vi "E7_28.vi"(4 "error in":T15, 7 "Command":T7) -> (0 "error out":T15, 3 "Response":T13)   [LabVIEW 2018]
uses:
  MOKO_LabViewLibrary/MokoLowLevel/MokoLowLovelControl/MLLC_Command.ctl
  MOKO_LabViewLibrary/MokoLowLevel/MokoLowLovelControl/MLLC_Error.ctl
  MOKO_LabViewLibrary/MokoLowLevel/MokoLowLovelControl/MLLC_Mode.ctl
  MOKO_LabViewLibrary/MokoLowLevel/MokoLowLovelControl/MLLC_Response.ctl
  MOKO_LabViewLibrary/MokoLowLevel/MokoLowLovelControl/MLLC_DriverName.ctl
  MOKO_LabViewLibrary/MokoLowLevel/MokoLowLovelControl/MLLC_ResponseInit.ctl
  MOKO_LabViewLibrary/MokoLowLevel/MokoLowLovelControl/MLLC_ErrorCode.ctl
  MOKO_LabViewLibrary/MokoLowLevel/MokoLowLovelControl/MLLC_Request.ctl
  MOKO_LabViewLibrary/MokoLowLevel/MokoLowLovelControl/MLLC_ConnectCluster.ctl
  MOKO_LabViewLibrary/MokoLowLevel/MokoLowLovelControl/MLLC_InterfaceType.ctl
  MOKO_LabViewLibrary/MokoLowLevel/MokoLowLovelControl/MLLC_OpenedSession.ctl
  MOKO_LabViewLibrary/MokoLowLevel/MokoLowLovelControl/MLLC_InterfaceSettings.ctl
  MOKO_LabViewLibrary/MokoLowLevel/MokoLowLovelControl/MLLC_InterfaceKind.ctl
  data/E7_28_DATA.ctl
  MOKO_LabViewLibrary/MokoLowLevel/MokoLowLovelControl/MLLC_Rs232Settings.ctl
panel:
  in  "Settings":T9={"Data"={"Connect"={"InterfaceType"=enum."VISA", "OpenedSession"="", "InterfaceSettings"={"Interface"=enum."RS232", "EOS 4 read"=enum."LF (\\n)", "EOS 4 write"=enum."LF (\\n)", "TMO, ms"=10000, "Sett"=variant(cluster{"Baud Rate":u32, "Data Bits":u16, "Parity":u16, "Stop Bits":u16, "Flow Control":u16, "Eho":bool} {"Baud Rate"=75, "Data Bits"=0, "Parity"=0, "Stop Bits"=0, "Flow Control"=0, "Eho"=FALSE})}}, "Cluster"={"flags"="", "freq"=0, "z"=0.0, "f"=0}, "Delay, ms"=100}, "Saved Data"=variant}
  in  "Request":T10="init"
  in  "Error Code":T8=5422
  in  "ResponseInit":T11="Є@E728"
  in  "Driver Name":T12="E7_28"
  in  "Mode":T14=enum."Check"
  # "E7-28"
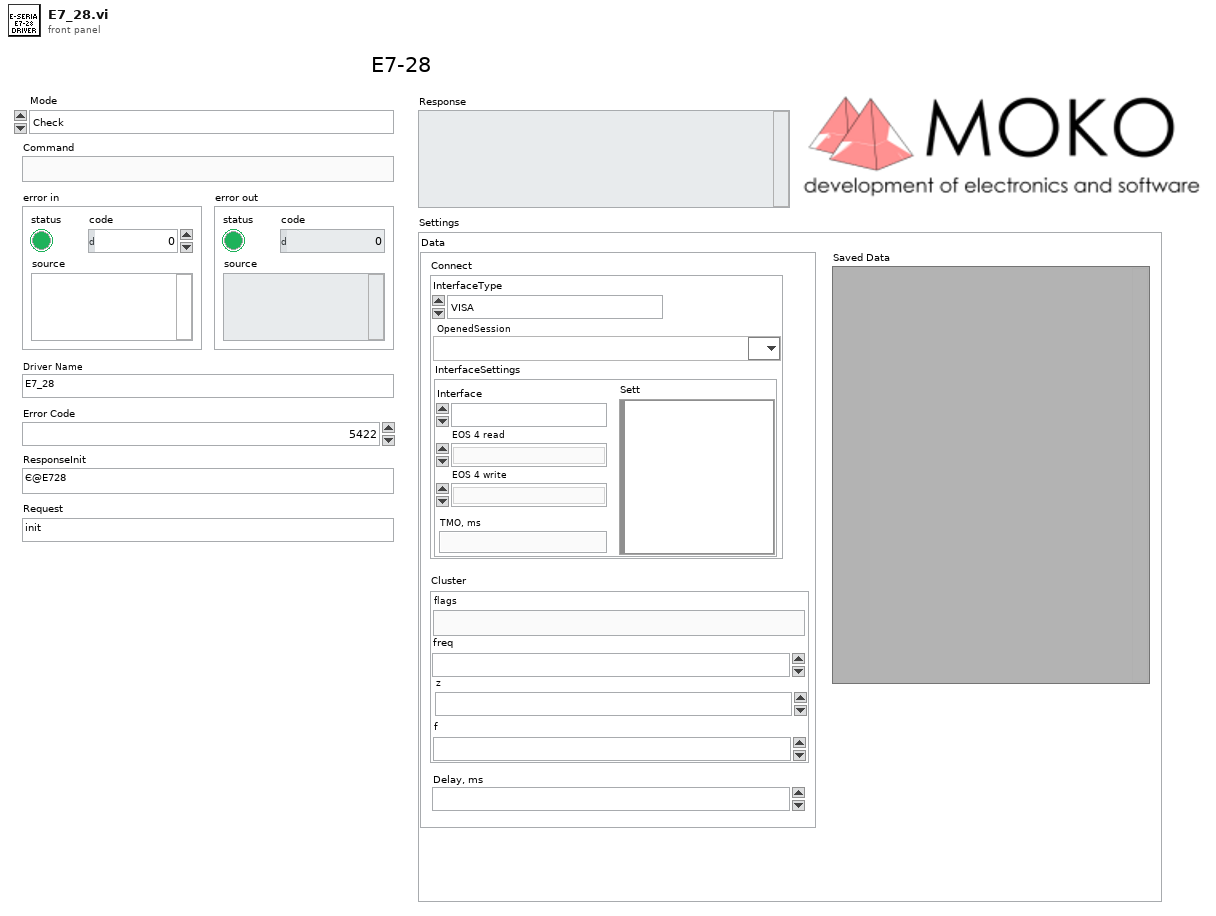
[diagram p1: front panel]
types:
  T1 = typedef "MLLC_ConnectCluster.ctl" = cluster{"InterfaceType":T2, "OpenedSession":T3, "InterfaceSettings":T4}
  T2 = typedef "MLLC_InterfaceType.ctl" = enum16{"VISA", "Prologix USB-GPIB"}
  T3 = typedef "MLLC_OpenedSession.ctl" = refnum<visa-resource-name>
  T4 = typedef "MLLC_InterfaceSettings.ctl" = cluster{"Interface":T5, "EOS 4 read":enum16{"Default (=EOS 4 write)", "CR (\\r)", "LF (\\n)", "None"}, "EOS 4 write":enum16{"CR+LF (\\r\\n)", "CR (\\r)", "LF (\\n)", "None"}, "TMO, ms":i32, "Sett":variant}
  T5 = typedef "MLLC_InterfaceKind.ctl" = enum16{"RS232", "GPIB", "USB", "Ethernet", "another"}
  T6 = typedef "E7_28_DATA.ctl" = cluster{"flags":T7, "freq":T8, "z":dbl, "f":T8}
  T7 = typedef "MLLC_Command.ctl" = string
  T8 = typedef "MLLC_ErrorCode.ctl" = u32
  T9 = cluster{"Data":cluster{"Connect":T1, "Cluster":T6, "Delay, ms":T8}, "Saved Data":variant}
  T10 = typedef "MLLC_Request.ctl" = string
  T11 = typedef "MLLC_ResponseInit.ctl" = string
  T12 = typedef "MLLC_DriverName.ctl" = string
  T13 = typedef "MLLC_Response.ctl" = string
  T14 = typedef "MLLC_Mode.ctl" = enum16{"get", "set", "close", "Init", "Check"}
  T15 = typedef "MLLC_Error.ctl" = errorcluster
  T16 = cluster{"Connect":T1, "Cluster":T6, "Delay, ms":T8}
  T17 = typedef "MLLC_Rs232Settings.ctl" = cluster{"Baud Rate":u32, "Data Bits":u16, "Parity":u16, "Stop Bits":u16, "Flow Control":u16, "Eho":bool, "Address":dbl}
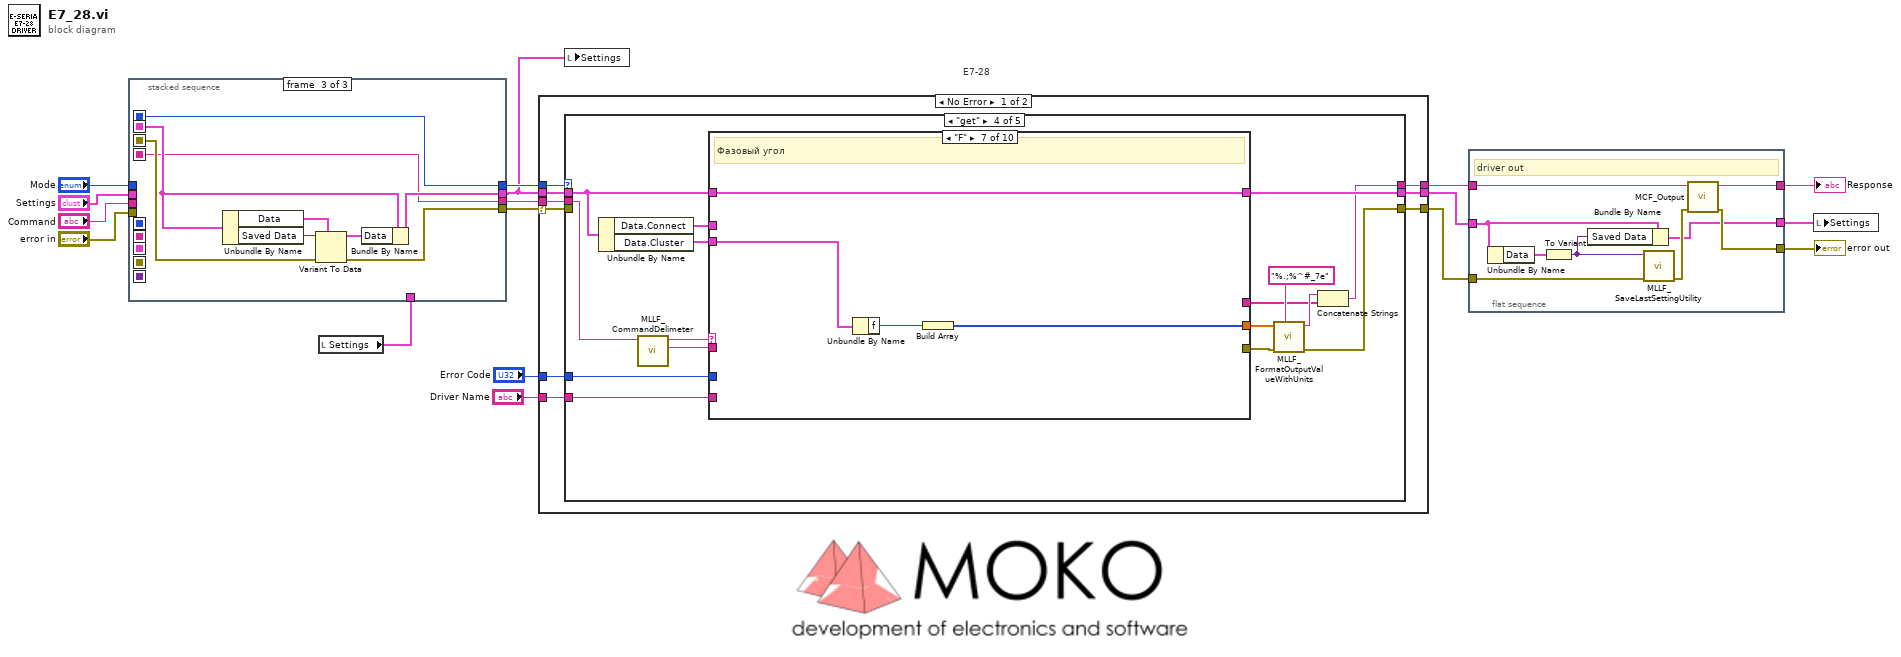
[diagram p0: block diagram]
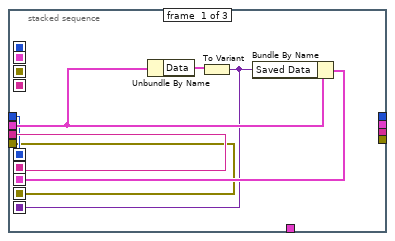
[diagram p2: hidden frame]
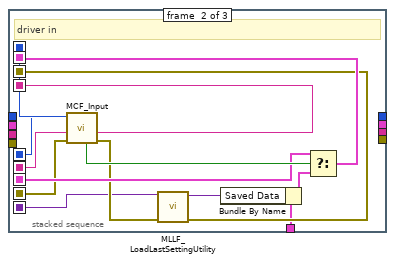
[diagram p3: hidden frame]
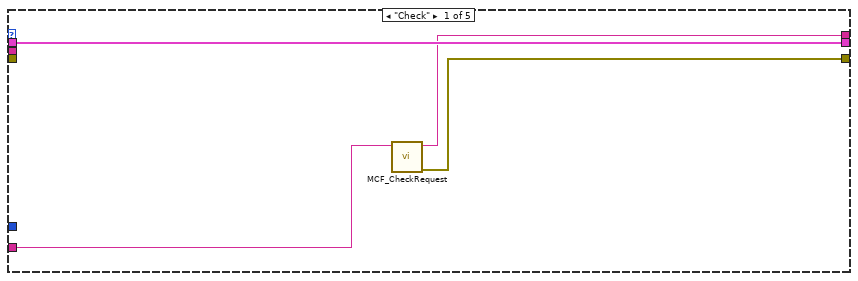
[diagram p4: hidden frame]
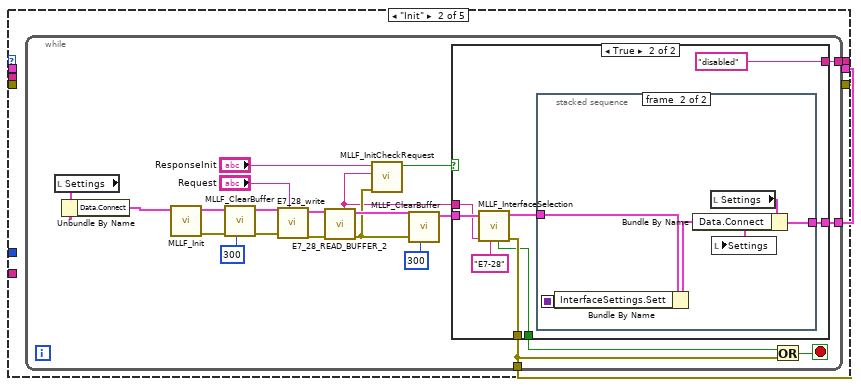
[diagram p5: hidden frame]
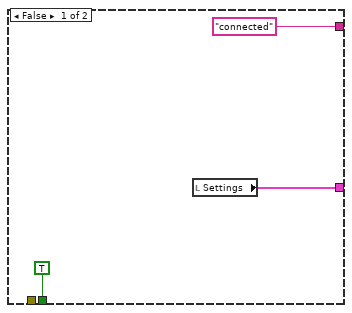
[diagram p6: hidden frame]
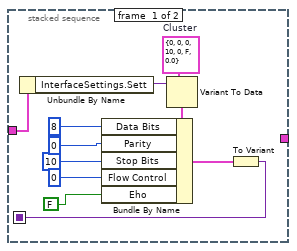
[diagram p7: hidden frame]
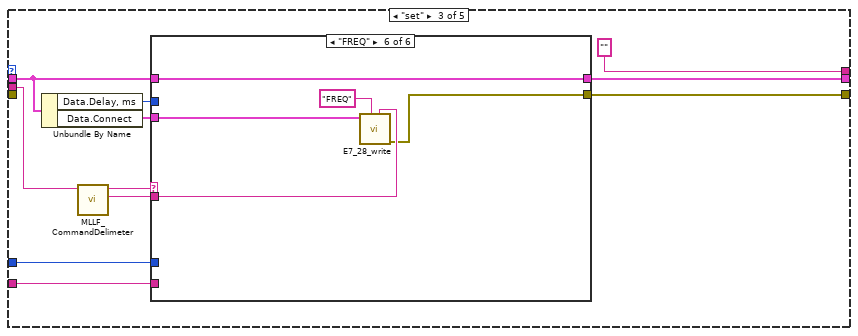
[diagram p8: hidden frame]
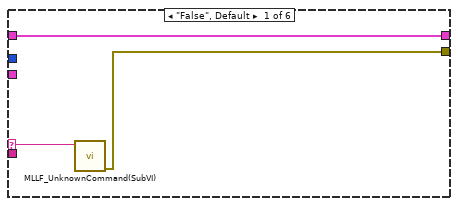
[diagram p9: hidden frame]
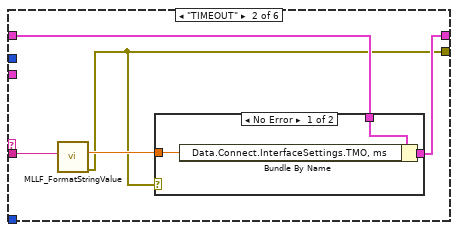
[diagram p10: hidden frame]
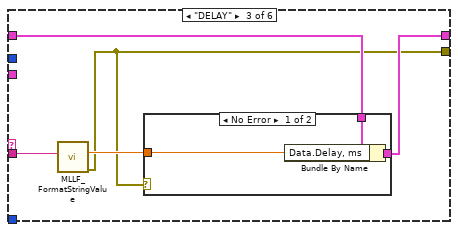
[diagram p12: hidden frame]
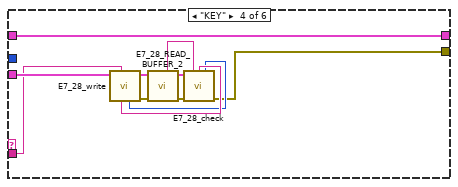
[diagram p14: hidden frame]
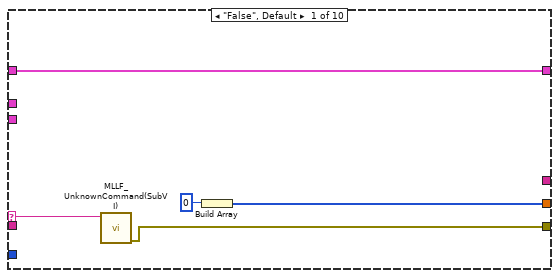
[diagram p16: hidden frame]
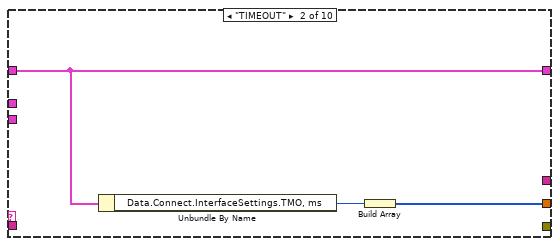
[diagram p17: hidden frame]
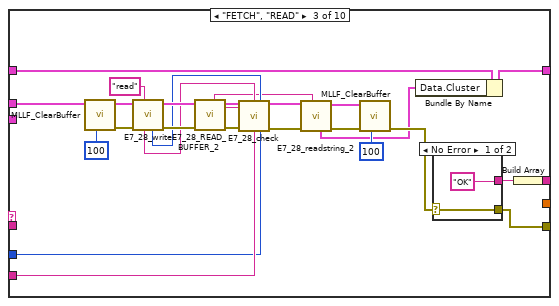
[diagram p18: hidden frame]
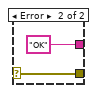
[diagram p19: hidden frame]
diagram:
  # "E7-28"
  n1 = local read "Settings"() -> (w7:T9)
  n2 = stacked-sequence {
    seq-local: [w20 _ _] -> [_ w36 _]
    seq-local: [w19 _ _] -> [_ w37 _]
    seq-local: [w22 _ _] -> [_ w32 _]
    seq-local: [w18 _ _] -> [_ w31 _]
    seq-local: [w21 _ _] -> [_ w27 _]
    seq-local: [_ w28 _] -> [_ _ w44]
    seq-local: [_ w38 _] -> [_ _ w41]
    seq-local: [_ w35 _] -> [_ _ w40]
    seq-local: [_ w34 _] -> [_ _ w45]
    tunnel: "Command" -> [w20 _ _]
    tunnel: "Mode" -> [w19 _ _]
    tunnel: "error in" -> [w18 _ _]
    tunnel: "Settings" -> [w23 _ _]
    tunnel: w7 -> [_ w26 _]
    tunnel: [_ _ w40] -> w9
    tunnel: [_ _ w43] -> w10
    tunnel: [_ _ w42] -> w8
    tunnel: [_ _ w41] -> w11
    frame #0 {
      n3 = Unbundle By Name(w23) -> ("Data"=w24:T16)
      n4 = To Variant(anything=w24) -> (Variant=w21:variant)
      n5 = Bundle By Name(cluster=w23, "Saved Data"=w21) -> (w22:T9)
    }
    frame #1 {
      # "driver in"
      n6 = call "MCF_Input.vi"("Error In"=w31, "Command in"=w36, "Mode in"=w37) -> ("Error Out"=w30:errorcluster, "Command out"=w35:string, "Mode out"=w38:T14, "Boolean"=w33:bool)  [unwired: 5 in]
      n7 = call "MLLF_LoadLastSettingUtility.vi"("Error In"=w30, "Save data in"=w27) -> ("Error Out"=w28:errorcluster, "Save data out"=w25:variant)  [unwired: 8 in]
      n8 = Bundle By Name(cluster=w26, "Saved Data"=w25) -> (w29:T9)
      n9 = Select(t=w32, s=w33, f=w29) -> (s? t:f=w34:T9)
    }
    frame #2 {
      n10 = Unbundle By Name(w45) -> ("Data"=w46:T16, "Saved Data"=w39:variant)
      n11 = Variant To Data(error in=w44, type=w46, Variant=w39) -> (data=w47:T16, error out=w42:errorcluster)
      n12 = Bundle By Name(cluster=w45, "Data"=w47) -> (w43:T9)
    }
  }
  n13 = case shown="No Error" w8 {
    selector: w8 -> [w52 w267]
    tunnel: [w54 w267] -> w4
    tunnel: w11 -> [w56 _]
    tunnel: [w55 "" ("String")] -> w6
    tunnel: w9 -> [w53 _]
    tunnel: w10 -> [w49 w266]
    tunnel: "Error Code" -> [w51 _]
    tunnel: "Driver Name" -> [w50 _]
    tunnel: [w48 w266] -> w5
    frame No Error {
      n14 = case shown="\"get\"" w56 {
        tunnel: [w59 w63 "" ("String") w163 _] -> w55
        tunnel: [w58 w61 w113 w162 w263] -> w54
        tunnel: w53 -> [_ _ w116 w166 _]
        tunnel: w52 -> [_ _ _ _ _]
        tunnel: w51 -> [_ _ w123 w175 _]
        tunnel: w50 -> [w57 _ w120 w174 _]
        tunnel: w49 -> [w60 _ w122 w177 w262]
        tunnel: [w60 w62 w121 w176 w262] -> w48
        frame "Check" {
          n15 = call "MCF_CheckRequest.vi"("Driver Name"=w57) -> ("Error Out"=w58:errorcluster, "Output String"=w59:string)  [unwired: 9 in]
        }
        frame "Init" {
          n16 = while {
            tunnel: [w83] -> w61
            tunnel: [w66] -> w63
            tunnel: [w65] -> w62
            stop <- w82 stop-if-true
            n17 = local read "Settings"() -> (w85:T9)
            n18 = Unbundle By Name(w85) -> ("Data.Connect"=w84:T1)
            n19 = call "MLLF_Init.vi"("DriverConnect in"=w84) -> ("Error Out"=w77:errorcluster, "DriverConnect out"=w78:T1)  [unwired: 7 in]
            n20 = call "MLLF_ClearBuffer.vi"("Timeout(default = 300 ms)"=u32 300 ("Timeout"), "Error In"=w77, "DriverConnect in"=w78) -> ("Error Out"=w75:errorcluster, "DriverConnect out"=w76:T1)  [unwired: 5 in, 1 out]
            n21 = call "E7_28_write.vi"("Command"="Request", "error in"=w75, "DriverConnect in"=w76) -> ("error out"=w80:T15, "DriverConnect out"=w79:T1)  [unwired: 5 in, 2 out]
            n22 = call "E7_28_READ_BUFFER_2.vi"("error in"=w80, "DriverConnect in"=w79) -> ("error out"=w69:T15, "DriverConnect out"=w72:T1, "String from device out"=w64:string)  [unwired: 7 in]
            n23 = call "MLLF_InitCheckRequest.vi"("error in (no error)"=w69, "Answer"=w64, "Response Init"="ResponseInit") -> ("Design"=w68:bool)  [unwired: 5 in, 3 out]
            n24 = call "MLLF_ClearBuffer.vi"("Timeout(default = 300 ms)"=u32 300 ("Timeout"), "Error In"=w69, "DriverConnect in"=w72) -> ("DriverConnect out"=w71:T1)  [unwired: 5 in, 2 out]
            n25 = case shown="True" w68 {
              tunnel: [_ w94] -> w83
              tunnel: [TRUE w90] -> w81
              tunnel: w71 -> [_ w96]
              tunnel: ["connected" "disabled"] -> w66
              tunnel: [w86 w91] -> w65
              tunnel: w64 -> [_ w89]
              frame False {
                n26 = local read "Settings"() -> (w86:T9)
              }
              frame True {
                n27 = call "MLLF_InterfaceSelection.vi"("Driver Name"="E7-28" ("String"), "Answer:"=w89, "DriverConnect in"=w96) -> ("error out"=w94:T15, "DriverConnect out"=w95:T1, "stop init?"=w90:bool)  [unwired: 4 in, 2 out]
                n28 = stacked-sequence {
                  seq-local: [w99 _] -> [_ w111]
                  tunnel: w95 -> [w97 w109]
                  tunnel: [_ w110] -> w91
                  frame #0 {
                    w106 = T17 {"Baud Rate"=0, "Data Bits"=0, "Parity"=0, "Stop Bits"=10, "Flow Control"=0, "Eho"=FALSE, "Address"=0.0}  # Cluster
                    n29 = Unbundle By Name(w97) -> ("InterfaceSettings.Sett"=w107:variant)
                    n30 = Variant To Data(type=w106, Variant=w107) -> (data=w105:T17)  [unwired: 1 in, 1 out]
                    n31 = Bundle By Name(cluster=w105, "Data Bits"=u16 8 ("Serial Settings:Data Bits"), "Parity"=u16 0 ("Serial Settings:Parity"), "Stop Bits"=u16 10 ("Serial Settings:Stop Bits"), "Flow Control"=u16 0 ("Serial Settings:Flow Control"), "Eho"=FALSE) -> (w100:T17)
                    n32 = To Variant(anything=w100) -> (Variant=w99:variant)
                  }
                  frame #1 {
                    n33 = Bundle By Name(cluster=w109, "InterfaceSettings.Sett"=w111) -> (w108:T1)
                    n34 = local read "Settings"() -> (w112:T9)
                    n35 = Bundle By Name(cluster=w112, "Data.Connect"=w108) -> (w110:T9)
                    n36 = local write "Settings"(w110) -> ()
                  }
                }
              }
            }
            n37 = Or(x=w81, y=w83) -> (x .or. y?=w82:bool)
          }
        }
        frame "set" {
          n38 = Unbundle By Name(w122) -> ("Data.Delay, ms"=w117:T8, "Data.Connect"=w118:T1)
          n39 = call "MLLF_CommandDelimeter.vi"("command with param"=w116) -> ("param 1"=w114:string, "command"=w115:string)  [unwired: 6 in, 3 out]
          n40 = case shown="\"FREQ\"" w115 {
            selector: w115 -> [w125 _ _ _ _ _]
            tunnel: w114 -> [_ w129 w138 w153 _ w158]
            tunnel: [w124 w127 w136 w145 _ w157] -> w113
            tunnel: w123 -> [_ _ _ _ _ _]
            tunnel: w122 -> [w126 w130 w139 w155 w156 w161]
            tunnel: [w126 w131 w140 w155 w156 w161] -> w121
            tunnel: w118 -> [_ _ _ w154 _ w160]
            tunnel: w120 -> [_ _ _ _ _ _]
            tunnel: w117 -> [_ _ _ _ _ _]
            frame "False", Default {
              n41 = call "MLLF_UnknownCommand(SubVI).vi"("Unknown command"=w125) -> ("error out"=w124:errorcluster)  [unwired: 10 in]
            }
            frame "TIMEOUT" {
              n42 = call "MLLF_FormatStringValue.vi"("String Value"=w129) -> ("error out"=w127:T15, "number"=w128:dbl)  [unwired: 8 in, 1 out]
              n43 = case shown="No Error" w127 {
                tunnel: [w134 w135] -> w131
                tunnel: w130 -> [w133 w135]
                tunnel: w128 -> [w132 _]
                frame No Error {
                  n44 = Bundle By Name(cluster=w133, "Data.Connect.InterfaceSettings.TMO, ms"=w132) -> (w134:T9)
                }
                frame Error {
                }
              }
            }
            frame "DELAY" {
              n45 = call "MLLF_FormatStringValue.vi"("String Value"=w138) -> ("error out"=w136:T15, "number"=w137:dbl)  [unwired: 8 in, 1 out]
              n46 = case shown="No Error" w136 {
                tunnel: [w143 w144] -> w140
                tunnel: w139 -> [w142 w144]
                tunnel: w137 -> [w141 _]
                frame No Error {
                  n47 = Bundle By Name(cluster=w142, "Data.Delay, ms"=w141) -> (w143:T9)
                }
                frame Error {
                }
              }
            }
            frame "KEY" {
              n48 = call "E7_28_write.vi"("Command"=w153, "DriverConnect in"=w154) -> ("error out"=w149:T15, "DriverConnect out"=w150:T1, "command HEX out"=w147:u16, "command string out"=w148:T7)  [unwired: 6 in]
              n49 = call "E7_28_READ_BUFFER_2.vi"("error in"=w149, "DriverConnect in"=w150) -> ("error out"=w151:T15, "DriverConnect out"=w152:T1, "String from device out"=w146:string)  [unwired: 7 in]
              n50 = call "E7_28_check.vi"("DriverConnect in"=w152, "String in"=w146, "command string in"=w148, "command HEX in"=w147, "error in"=w151) -> ("error out"=w145:T15)  [unwired: 9 in, 1 out]
            }
            frame "---------------------------------------------------------------------------------------" {
            }
            frame "FREQ" {
              n51 = call "E7_28_write.vi"("VALUE"=w158, "Command"="FREQ", "DriverConnect in"=w160) -> ("error out"=w157:T15)  [unwired: 5 in, 3 out]
            }
          }
        }
        frame "get" {
          n52 = Unbundle By Name(w177) -> ("Data.Connect"=w170:T1, "Data.Cluster"=w167:T6)
          n53 = call "MLLF_CommandDelimeter.vi"("command with param"=w166) -> ("param 1"=w164:string, "command"=w165:string)  [unwired: 6 in, 3 out]
          n54 = case shown="\"F\"" w165 {
            selector: w165 -> [w179 _ _ _ _ _ _ _ _ _]
            tunnel: w164 -> [_ _ _ _ _ _ _ _ _ _]
            tunnel: [w178 _ w195 _ _ _ _ _ _ _] -> w172
            tunnel: w175 -> [_ _ w200 _ _ _ _ _ _ _]
            tunnel: [w182 w185 w187 w216 w217 w221 w225 w234 w244 w256] -> w176
            tunnel: [w180 w183 _ _ w218 w222 w226 w236 w245 w257] -> w171
            tunnel: w170 -> [_ _ w205 _ _ _ _ _ _ _]
            tunnel: w174 -> [_ _ w201 _ _ _ _ _ _ _]
            tunnel: [_ _ w196 _ _ _ _ _ _ _] -> w168
            tunnel: w167 -> [_ _ _ _ w220 w224 w228 w240 w246 w259]
            tunnel: w177 -> [w182 w185 w188 w216 w217 w221 w225 w234 w244 w256]
            frame "False", Default {
              n55 = call "MLLF_UnknownCommand(SubVI).vi"("Unknown command"=w179) -> ("error out"=w178:errorcluster)  [unwired: 10 in]
              n56 = Build Array(0 ("TimeOut")) -> (w180:i32[])
            }
            frame "TIMEOUT" {
              n57 = Unbundle By Name(w185) -> ("Data.Connect.InterfaceSettings.TMO, ms"=w184:i32)
              n58 = Build Array(w184) -> (w183:i32[])
            }
            frame "FETCH", "READ" {
              n59 = call "MLLF_ClearBuffer.vi"("Timeout(default = 300 ms)"=u32 100 ("Timeout"), "DriverConnect in"=w205) -> ("Error Out"=w208:errorcluster, "DriverConnect out"=w209:T1)  [unwired: 6 in, 1 out]
              n60 = call "E7_28_write.vi"("Command"="read", "error in"=w208, "DriverConnect in"=w209) -> ("error out"=w211:T15, "DriverConnect out"=w210:T1, "command HEX out"=w198:u16, "command string out"=w199:T7)  [unwired: 5 in]
              n61 = call "E7_28_READ_BUFFER_2.vi"("error in"=w211, "DriverConnect in"=w210) -> ("error out"=w202:T15, "DriverConnect out"=w203:T1, "String from device out"=w192:string)  [unwired: 7 in]
              n62 = call "E7_28_check.vi"("DriverConnect in"=w203, "String in"=w192, "command string in"=w199, "command HEX in"=w198, "error in"=w202, "Driver Name"=w201, "Error Code"=w200) -> ("DriverConnect out"=w194:T1, "error out"=w193:T15)  [unwired: 7 in]
              n63 = call "E7_28_readstring_2.vi"("data string"=w192, "error in"=w193, "DriverConnect in"=w194) -> ("error out"=w190:T15, "DriverConnect out"=w191:T1, "Cluster 2"=w186:T6)  [unwired: 6 in]
              n64 = call "MLLF_ClearBuffer.vi"("Timeout(default = 300 ms)"=u32 100 ("Timeout"), "Error In"=w190, "DriverConnect in"=w191) -> ("Error Out"=w189:errorcluster)  [unwired: 5 in, 2 out]
              n65 = Bundle By Name(cluster=w188, "Data.Cluster"=w186) -> (w187:T9)
              n66 = case shown="No Error" w189 {
                selector: w189 -> [w213 w214]
                tunnel: [w213 w214] -> w195
                tunnel: ["OK" "OK"] -> w197
                frame No Error {
                }
                frame Error {
                }
              }
              n67 = Build Array(w197) -> (w196:string[])
            }
            frame "---------------------------------------------------------" {
            }
            frame "FREQ" {
              n68 = Unbundle By Name(w220) -> ("freq"=w219:T8)
              n69 = Build Array(w219) -> (w218:T8[])
            }
            frame "Z" {
              # "Модуль комплексного сопротивления, Z"
              n70 = Unbundle By Name(w224) -> ("z"=w223:dbl)
              n71 = Build Array(w223) -> (w222:dbl[])
            }
            frame "F" {
              # "Фазовый угол"
              n72 = Unbundle By Name(w228) -> ("f"=w227:T8)
              n73 = Build Array(w227) -> (w226:T8[])
            }
            frame "C" {
              # "Емкость С, Ф"
              n74 = Unbundle By Name(w240) -> ("freq"=w239:T8)
              n75 = Unbundle By Name(w240) -> ("z"=w243:dbl)
              n76 = Unbundle By Name(w240) -> ("f"=w230:T8)
              n77 = Divide(x=w230, y=57.2958) -> (x/y=w231:dbl)
              n78 = Sine(x=w231) -> (sin(x)=w242:dbl)
              n79 = Multiply(x=w243, y=w242) -> (x*y=w241:dbl)
              n80 = Multiply(x=w239, y=6.283185307179586) -> (x*y=w237:dbl)
              n81 = Multiply(x=w241, y=w237) -> (x*y=w235:dbl)
              n82 = Reciprocal(x=w235) -> (1/x=w233:dbl)
              n83 = Absolute Value(x=w233) -> (abs(x)=w232:dbl)
              n84 = Build Array(w232) -> (w236:dbl[])
            }
            frame "R", "Rs" {
              n85 = Unbundle By Name(w246) -> ("z"=w253:dbl)
              n86 = Unbundle By Name(w246) -> ("f"=w248:T8)
              n87 = Divide(x=w248, y=57.2958) -> (x/y=w247:dbl)
              n88 = Absolute Value(x=w253) -> (abs(x)=w252:dbl)
              n89 = Cosine(x=w247) -> (cos(x)=w251:dbl)
              n90 = Multiply(x=w252, y=w251) -> (x*y=w250:dbl)
              n91 = Build Array(w250) -> (w245:dbl[])
            }
            frame "D" {
              # "Фактор потерь, D"
              n92 = Unbundle By Name(w259) -> ("f"=w261:T8)
              n93 = Divide(x=w261, y=57.2958) -> (x/y=w258:dbl)
              n94 = Tangent(1:w258) -> (0:w255:dbl)
              n95 = Absolute Value(x=w255) -> (abs(x)=w254:dbl)
              n96 = Build Array(w254) -> (w257:dbl[])
            }
          }
          n97 = call "MLLF_FormatOutputValueWithUnits.vi"("Format"="%.;%^#_7e" ("format string"), "error in"=w172, "ValuesIn"=w171) -> ("error out"=w162:T15, "Result string"=w173:T7)  [unwired: 7 in]
          n98 = Concatenate Strings(w173, w168) -> (w163:string)
        }
        frame "close" {
          n99 = Unbundle By Name(w262) -> ("Data.Connect.OpenedSession"=w264:T3)
          n100 = VISA Close(VISA resource name=w264) -> (error out=w263:errorcluster)  [unwired: 1 in]
        }
      }
    }
    frame Error {
    }
  }
  n101 = local write "Settings"(w10) -> ()
  n102 = flat-sequence {
    tunnel: [w276] -> w3
    tunnel: [w275] -> w1
    tunnel: w6 -> [w274]
    tunnel: w4 -> [w273]
    tunnel: w5 -> [w270]
    tunnel: [w268] -> _
    tunnel: [w268] -> w2
    frame #0 {
      # "driver out"
      n103 = Unbundle By Name(w270) -> ("Data"=w269:T16)
      n104 = To Variant(anything=w269) -> (Variant=w271:variant)
      n105 = Bundle By Name(cluster=w270, "Saved Data"=w271) -> (w268:T9)
      n106 = call "MLLF_SaveLastSettingUtility.vi"("error in"=w273, "Saved Data"=w271) -> ("error out"=w272:T15)  [unwired: 8 in, 1 out]
      n107 = call "MCF_Output.vi"("Error In"=w272, "Input"=w274) -> ("Error Out"=w275:errorcluster, "Output"=w276:string)  [unwired: 8 in]
    }
  }
  n108 = local write "Settings"(w2) -> ()
  "error out" <- w1
  "Response" <- w3
